vi "Initialize jettl.vi"(6 "Self":refnum<data-value>, 8 "Self Alias":string, 9 "Caller":refnum<data-value>, 10 "Caller Alias":string) -> (3 "jettl Queue Actor out":refnum<class "jettl Queue Actor.lvclass">)   [LabVIEW 2021, in "jettl.lvlib" / "jettl Queue Actor.lvlib" / "jettl Queue Actor.lvclass"]
uses:
  jettl Queue Actor.lvclass
  jettl Queue Actor.lvclass/jettl Queue Actor.ctl
  State/Nominal State/Nominal State.lvclass
  C:/git/jettl/src/jettl/jettl Queue Actor/State/Nominal State/Nominal State.lvclass
  C:/git/jettl/src/jettl/jettl Queue Actor/State/State/State.lvclass
  Actor/Msg/Msg.lvclass
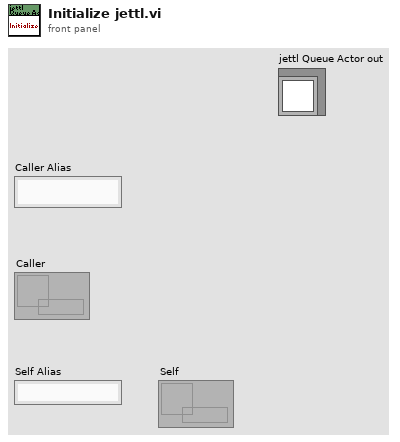
[diagram p1: front panel]
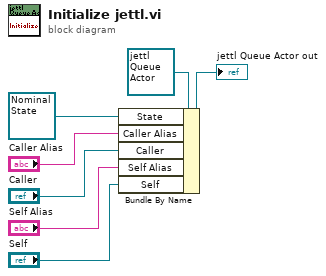
[diagram p0: block diagram]
diagram:
  n1 = Bundle By Name(cluster=refnum<class "jettl Queue Actor.lvclass"> refnum ("Self Actor in"), "State"=refnum<class "Nominal State.lvclass"> refnum ("LVCAM.lvlib:Msging Self Actor State.lvclass"), "Caller Alias"="Caller Alias", "Caller"="Caller", "Self Alias"="Self Alias", "Self"="Self") -> (→"jettl Queue Actor out":refnum<class "jettl Queue Actor.lvclass">)
